vi "Test_Execute Measurement.vi"   [LabVIEW 2020, in "Measurement Client Wrapper.lvclass"]
uses:
  Measurement Client Wrapper.lvclass
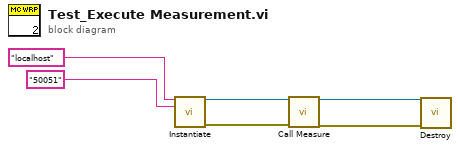
[diagram p0: block diagram]
diagram:
  n1 = call "Instantiate.vi"("location"="localhost", "insecurePort"="50051") -> ("Measurement Client Wrapper out"=w4:refnum<class "Measurement Client Wrapper.lvclass">, "error out"=w1:errorcluster)  [unwired: 12 in]
  n2 = call "Call Measure.vi"("Measurement Client Wrapper in"=w4, "error in (no error)"=w1) -> ("Measurement Client Wrapper out"=w3:refnum<class "Measurement Client Wrapper.lvclass">, "error out"=w2:errorcluster)  [unwired: 11 in, 1 out]
  n3 = call "Destroy.vi"("Measurement Client Wrapper in"=w3, "error in"=w2) -> ()  [unwired: 12 in, 2 out]
